vi "Time.Calc Next Scheduled Event.vi"(7 "IntervalSec(F)/Timeof Day(T)":bool, 10 "Seconds":dbl=3600.0, 11 "ScheduleTimeOfDay":timestamp=timestamp(-25200 s since 1904-01-01) format="%<%I:%M %p>T") -> (2 "Seconds to Wait":dbl, 3 "Sched Time":timestamp format="%<%I:%M:%S %p\n%x>T")   [LabVIEW 2018]
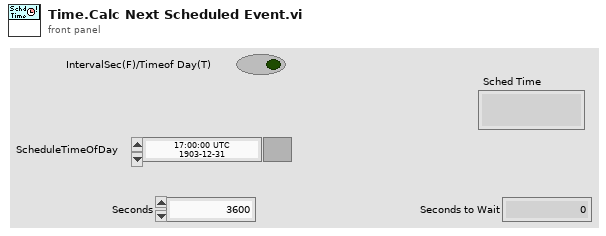
[diagram p1: front panel]
types:
  T1 = typedef "LVDateTimeRec.ctl" = cluster{"fractional second":dbl, "second":i32, "minute":i32, "hour":i32, "day of month":i32, "month":i32, "year":i32, "day of week":i32, "day of year":i32, "DST":i32}
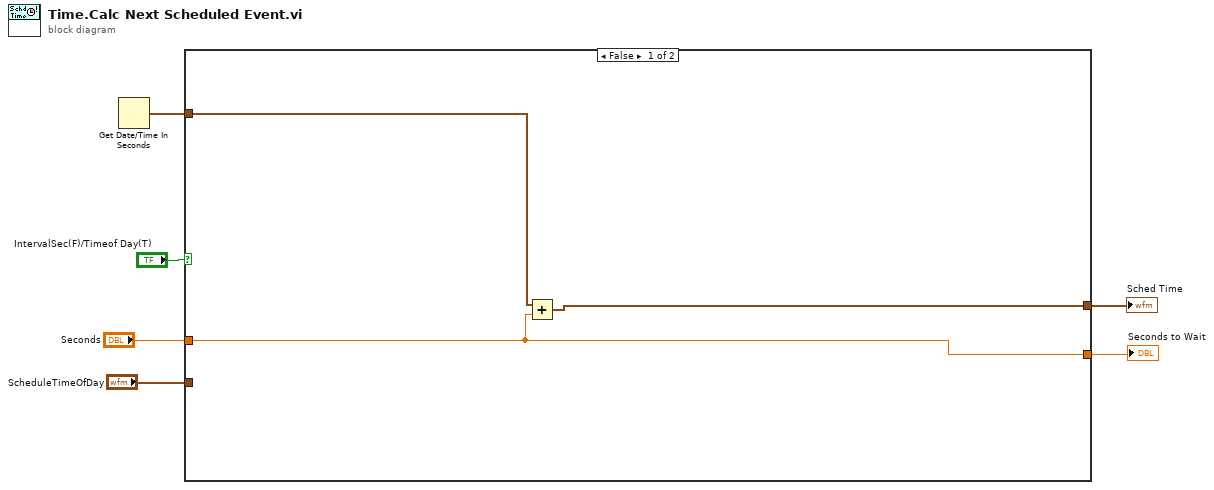
[diagram p0: block diagram]
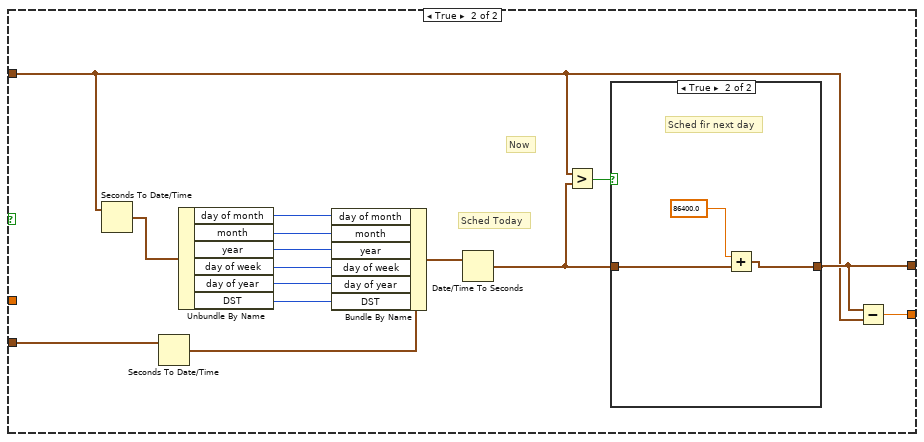
[diagram p2: hidden frame]
diagram:
  n1 = Get Date/Time In Seconds() -> (seconds since 1Jan1904=w4:timestamp)
  n2 = case shown="False" "IntervalSec(F)/Timeof Day(T)" {
    tunnel: [w8 w13] -> w6
    tunnel: [w7 w12] -> w5
    tunnel: w4 -> [w9 w11]
    tunnel: "Seconds" -> [w8 _]
    tunnel: "ScheduleTimeOfDay" -> [_ w10]
    frame False {
      n3 = Add(x=w9, y=w8) -> (x+y=w7:timestamp)
    }
    frame True {
      # "Sched Today"
      # "Now"
      n4 = Seconds To Date/Time(time stamp (now)=w11) -> (date time rec=w24:T1)  [unwired: 1 in]
      n5 = Seconds To Date/Time(time stamp (now)=w10) -> (date time rec=w14:T1)  [unwired: 1 in]
      n6 = Unbundle By Name(w24) -> ("day of month"=w23:i32, "month"=w22:i32, "year"=w21:i32, "day of week"=w20:i32, "day of year"=w19:i32, "DST"=w18:i32)
      n7 = Bundle By Name(cluster=w14, "day of month"=w23, "month"=w22, "year"=w21, "day of week"=w20, "day of year"=w19, "DST"=w18) -> (w17:T1)
      n8 = Date/Time To Seconds(2:w17) -> (0:w15:timestamp)  [unwired: 1 in]
      n9 = Greater?(x=w11, y=w15) -> (0:w16:bool)
      n10 = case shown="True" w16 {
        tunnel: w15 -> [w25 w28]
        tunnel: [w25 w26] -> w12
        frame False {
          # "Keep Today"
        }
        frame True {
          # "Sched fir next day"
          n11 = Add(x=86400.0, y=w28) -> (x+y=w26:timestamp)
        }
      }
      n12 = Subtract(x=w12, y=w11) -> (x-y=w13:dbl)
    }
  }
  "Seconds to Wait" <- w6
  "Sched Time" <- w5
